vi "Create and Start gRPC Server.vi"(5 "Server Key File (.key)":path, 7 "Server Certificate File (.crt)":path, 8 "error in (no error)":errorcluster, 10 "Server Address":string="localhost:15882", 11 "CIFLauncher in":refnum<class "CIFLauncher.lvclass">) -> (0 "error out":errorcluster, 3 "CIFLauncher out":refnum<class "CIFLauncher.lvclass">)   [LabVIEW 2021, in "CIFLauncher.lvclass"]
uses:
  CIFLauncher.lvclass
  CIFLauncher.lvclass/CIFLauncher.ctl
  <vilib>/gRPC/LabVIEW gRPC Servicer/Servicer/Servicer.lvclass
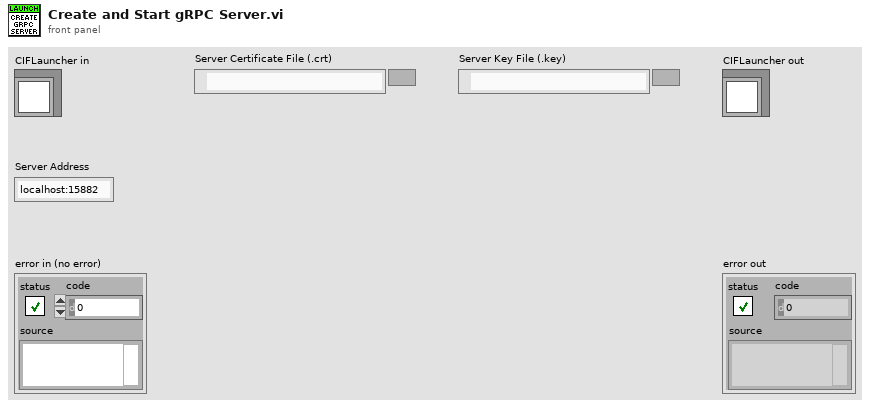
[diagram p1: front panel]
types:
  T1 = typedef "grpc-lvsupport-release.lvlib/grpcId.ctl" = u64
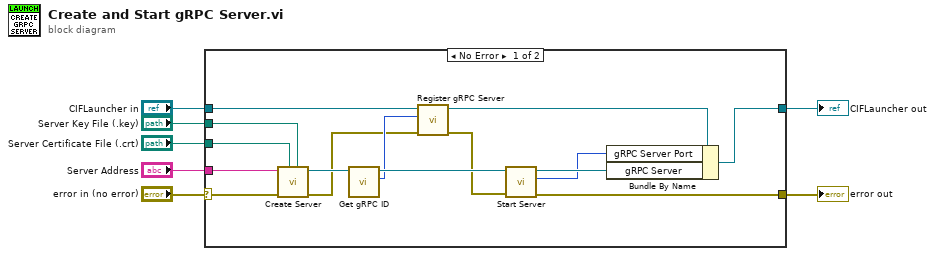
[diagram p0: block diagram]
diagram:
  n1 = case shown="No Error" "error in (no error)" {
    selector: "error in (no error)" -> [w18 w24]
    tunnel: [w17 w24] -> w4
    tunnel: [w14 w23] -> w1
    tunnel: "CIFLauncher in" -> [w12 w23]
    tunnel: "Server Certificate File (.crt)" -> [w20 _]
    tunnel: "Server Key File (.key)" -> [w19 _]
    tunnel: "Server Address" -> [w13 _]
    frame No Error {
      n2 = call <vilib>:"Create Server.vi"("Server Key File (.key)"=w19, "Server Certificate File (.crt)"=w20, "error in"=w18, "Server Address"=w13) -> ("error out"=w10:errorcluster, "gRPC Server out"=w22:refnum<class "Servicer.lvclass">)  [unwired: 6 in]
      n3 = call <vilib>:"Get gRPC ID.vi"("OOP Server in"=w22) -> ("gRPC ID"=w11:T1, "OOP Server out"=w21:refnum<class "Servicer.lvclass">)  [unwired: 9 in]
      n4 = call "Register gRPC Server.vi"("error in (no error)"=w10, "gRPC ID"=w11, "CIFLauncher in"=w12) -> ("error out"=w8:errorcluster, "CIFLauncher out"=w9:refnum<class "CIFLauncher.lvclass">)  [unwired: 7 in]
      n5 = call <vilib>:"Start Server.vi"("error in"=w8, "gRPC Server in"=w21) -> ("error out"=w17:errorcluster, "Listening Port"=w15:i32, "gRPC Server out"=w16:refnum<class "Servicer.lvclass">)  [unwired: 7 in]
      n6 = Bundle By Name(cluster=w9, "gRPC Server Port"=w15, "gRPC Server"=w16) -> (w14:refnum<class "CIFLauncher.lvclass">)
    }
    frame Error {
    }
  }
  "error out" <- w4
  "CIFLauncher out" <- w1
